vi "UDP Data Link - Driver Utilities - Get RT Data Refs.vi"(8 "error in (no error)":errorcluster, 11 "Device Ref in":T4 format="%.0x") -> (0 "error out":errorcluster, 1 "Rx Data Refs":T3 {"Block Data Refs"."Data Reference" format="%.0x"}, 2 "Tx Data Refs":T3 {"Block Data Refs"."Data Reference" format="%.0x"}, 3 "Device Ref out":T4=18446744073709551615 format="%.0x", 5 "Rx FIFO Timeout":u32, 7 "Rx FIFO Polling Rate":u32)   [LabVIEW 2012, in "UDP Data Link Engine.lvlib"]
uses:
  UDP Data Link Engine.lvlib
  <vilib>/NI Veristand/Custom Device API/Custom Device Item Ref.ctl
  <vilib>/NI Veristand/Custom Device API/Block Data Reference.ctl
  <vilib>/NI Veristand/Custom Device API/Data Reference.ctl
  <vilib>/NI Veristand/Custom Device API/Data Access Type.ctl
  Shared/UDP Data Link Global.vi
  <vilib>/NI Veristand/Custom Device API/Get Item Property (U16).vi
  <vilib>/NI Veristand/Custom Device API/Get Item Property (Dependent Node Pointer).vi
  <vilib>/NI Veristand/Custom Device Tools/Custom Device Utility Library/Custom Device Utility Library.lvlib
  Shared/UDP Data Link Shared.lvlib
  <vilib>/NI Veristand/Custom Device API/Custom Device API.lvlib
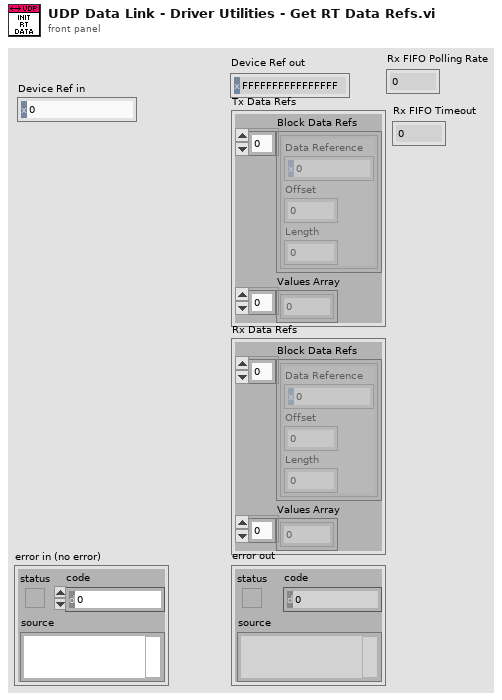
[diagram p1: front panel]
types:
  T1 = typedef "Custom Device API.lvlib/Block Data Reference.ctl" = cluster{"Data Reference":T2, "Offset":i32, "Length":i32}
  T2 = typedef "Custom Device API.lvlib/Data Reference.ctl" = i32
  T3 = cluster{"Block Data Refs":T1[], "Values Array":dbl[]}
  T4 = typedef "Custom Device API.lvlib/Custom Device Item Ref.ctl" = u64
  T5 = typedef "Custom Device API.lvlib/Data Access Type.ctl" = enum16{"Read", "Write"}
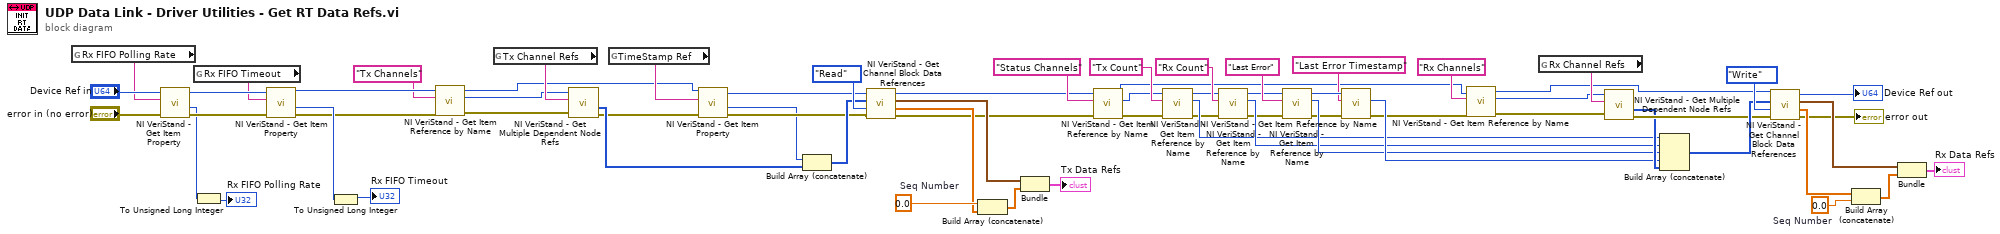
[diagram p0: block diagram]
diagram:
  w65 = 0.0  # Seq Number
  w46 = 0.0  # Seq Number
  n1 = global read "UDP Data Link Global.vi" "Rx FIFO Polling Rate"() -> (w29:string)
  n2 = call-poly <vilib>:"NI VeriStand - Get Item Property.vi"("error in (no error)"="error in (no error)", "Property Name"=w29, "Item Ref in"="Device Ref in") -> ("error out"=w28:errorcluster, "Value"=w25:u16, "Item Ref out"=w27:T4)  [unwired: 5 in, 1 out]
  n3 = global read "UDP Data Link Global.vi" "Rx FIFO Timeout"() -> (w26:string)
  n4 = To Unsigned Long Integer(number=w25) -> (unsigned 32bit integer=→"Rx FIFO Polling Rate":u32)
  n5 = call-poly <vilib>:"NI VeriStand - Get Item Property.vi"("error in (no error)"=w28, "Property Name"=w26, "Item Ref in"=w27) -> ("error out"=w23:errorcluster, "Value"=w24:u16, "Item Ref out"=w21:T4)  [unwired: 5 in, 1 out]
  n6 = To Unsigned Long Integer(number=w24) -> (unsigned 32bit integer=→"Rx FIFO Timeout":u32)
  n7 = call <vilib>:"NI VeriStand - Get Item Reference by Name.vi"("error in (no error)"=w23, "Item Name"="Tx Channels", "Parent Ref in"=w21) -> ("error out"=w22:errorcluster, "Item Ref"=w19:T4, "Parent Ref out"=w20:T4)  [unwired: 5 in, 1 out]
  n8 = global read "UDP Data Link Global.vi" "Tx Channel Refs"() -> (w35:string)
  n9 = call <vilib>:"NI VeriStand - Get Multiple Dependent Node Refs.vi"("error in (no error)"=w22, "Base Property Name"=w35, "Item Ref in"=w19) -> ("error out"=w36:errorcluster, "Dependent Node Refs"=w39:T4[])  [unwired: 6 in, 1 out]
  n10 = global read "UDP Data Link Global.vi" "TimeStamp Ref"() -> (w37:string)
  n11 = call-poly <vilib>:"NI VeriStand - Get Item Property.vi"("error in (no error)"=w36, "Property Name"=w37, "Item Ref in"=w20) -> ("error out"=w40:errorcluster, "Dependent Node Ref"=w38:T4, "Item Ref out"=w42:T4)  [unwired: 5 in, 1 out]
  n12 = Build Array (concatenate)(w38, w39) -> (w41:T4[])
  n13 = call <vilib>:"NI VeriStand - Get Channel Block Data References.vi"("error in (no error)"=w40, "Access"=Data_Access_Type."Read", "Channel Refs"=w41, "Device Ref in"=w42) -> ("error out"=w8:errorcluster, "Values Array"=w45:dbl[], "Block Data Refs"=w44:T1[], "Device Ref out"=w4:T4)  [unwired: 4 in]
  n14 = Build Array (concatenate)(w46, w45) -> (w47:dbl[])
  n15 = Bundle("Block Data Refs"=w44, w47) -> (→"Tx Data Refs":cluster{"Block Data Refs":T1[], dbl[]})  [unwired: 1 in]
  n16 = call <vilib>:"NI VeriStand - Get Item Reference by Name.vi"("error in (no error)"=w8, "Item Name"="Status Channels", "Parent Ref in"=w4) -> ("error out"=w7:errorcluster, "Item Ref"=w5:T4, "Parent Ref out"=w3:T4)  [unwired: 5 in, 1 out]
  n17 = call <vilib>:"NI VeriStand - Get Item Reference by Name.vi"("error in (no error)"=w7, "Item Name"="Tx Count", "Parent Ref in"=w5) -> ("error out"=w12:errorcluster, "Item Ref"=w56:T4, "Parent Ref out"=w49:T4)  [unwired: 5 in, 1 out]
  n18 = call <vilib>:"NI VeriStand - Get Item Reference by Name.vi"("error in (no error)"=w12, "Item Name"="Rx Count", "Parent Ref in"=w49) -> ("error out"=w11:errorcluster, "Item Ref"=w57:T4, "Parent Ref out"=w51:T4)  [unwired: 5 in, 1 out]
  n19 = call <vilib>:"NI VeriStand - Get Item Reference by Name.vi"("error in (no error)"=w11, "Item Name"="Last Error", "Parent Ref in"=w51) -> ("error out"=w10:errorcluster, "Item Ref"=w58:T4, "Parent Ref out"=w54:T4)  [unwired: 5 in, 1 out]
  n20 = call <vilib>:"NI VeriStand - Get Item Reference by Name.vi"("error in (no error)"=w10, "Item Name"="Last Error Timestamp", "Parent Ref in"=w54) -> ("error out"=w9:errorcluster, "Item Ref"=w59:T4)  [unwired: 5 in, 2 out]
  n21 = call <vilib>:"NI VeriStand - Get Item Reference by Name.vi"("error in (no error)"=w9, "Item Name"="Rx Channels", "Parent Ref in"=w3) -> ("error out"=w17:errorcluster, "Item Ref"=w15:T4, "Parent Ref out"=w16:T4)  [unwired: 5 in, 1 out]
  n22 = global read "UDP Data Link Global.vi" "Rx Channel Refs"() -> (w55:string)
  n23 = call <vilib>:"NI VeriStand - Get Multiple Dependent Node Refs.vi"("error in (no error)"=w17, "Base Property Name"=w55, "Item Ref in"=w15) -> ("error out"=w61:errorcluster, "Dependent Node Refs"=w60:T4[])  [unwired: 6 in, 1 out]
  n24 = Build Array (concatenate)(w56, w57, w58, w59, w60) -> (w62:T4[])
  n25 = call <vilib>:"NI VeriStand - Get Channel Block Data References.vi"("error in (no error)"=w61, "Access"=Data_Access_Type."Write", "Channel Refs"=w62, "Device Ref in"=w16) -> ("error out"=→"error out":errorcluster, "Values Array"=w64:dbl[], "Block Data Refs"=w66:T1[], "Device Ref out"=→"Device Ref out":T4)  [unwired: 4 in]
  n26 = Build Array (concatenate)(w64, w65) -> (w67:dbl[])
  n27 = Bundle("Block Data Refs"=w66, w67) -> (→"Rx Data Refs":cluster{"Block Data Refs":T1[], dbl[]})  [unwired: 1 in]
